vi "pitchrolldistance.vi"(11 "input":dbl[](array[numeric])) -> (3 "A * B 2":T1)   [LabVIEW 2015]
uses:
  <vilib>/Analysis/Matrix/Datatypes/RealMatrix.ctl
  <vilib>/Analysis/baseanly.llb/Unit Vector (DBL).vi
  <vilib>/Analysis/Matrix/Numeric/Conversions/Array To Matrix - RA2.vi
  <vilib>/Analysis/Matrix/Numeric/Conversions/Array To Matrix - RA.vi
  <vilib>/Analysis/Matrix/Numeric/Subtract/Subtract - RM,RM.vi
  <vilib>/Analysis/Matrix/Numeric/Multiply/Multiply - RM,RM.vi
  <vilib>/Analysis/NI_AALPro.lvlib
  <vilib>/Analysis/Matrix/NI_Matrix.lvlib
  <vilib>/Analysis/NI_AALBase.lvlib
panel:
  out "Position points":i32[][](array[numeric])
  out "Unit Vector":dbl[](array[numeric]) format="%0.2f"
  out "A * B":T1
  out "Real Matrix (Column Vector)":T1
  out "Real Matrix":T1
  out "x-y 2":dbl[](array[numeric])
  out "x-y":dbl[](array[numeric])
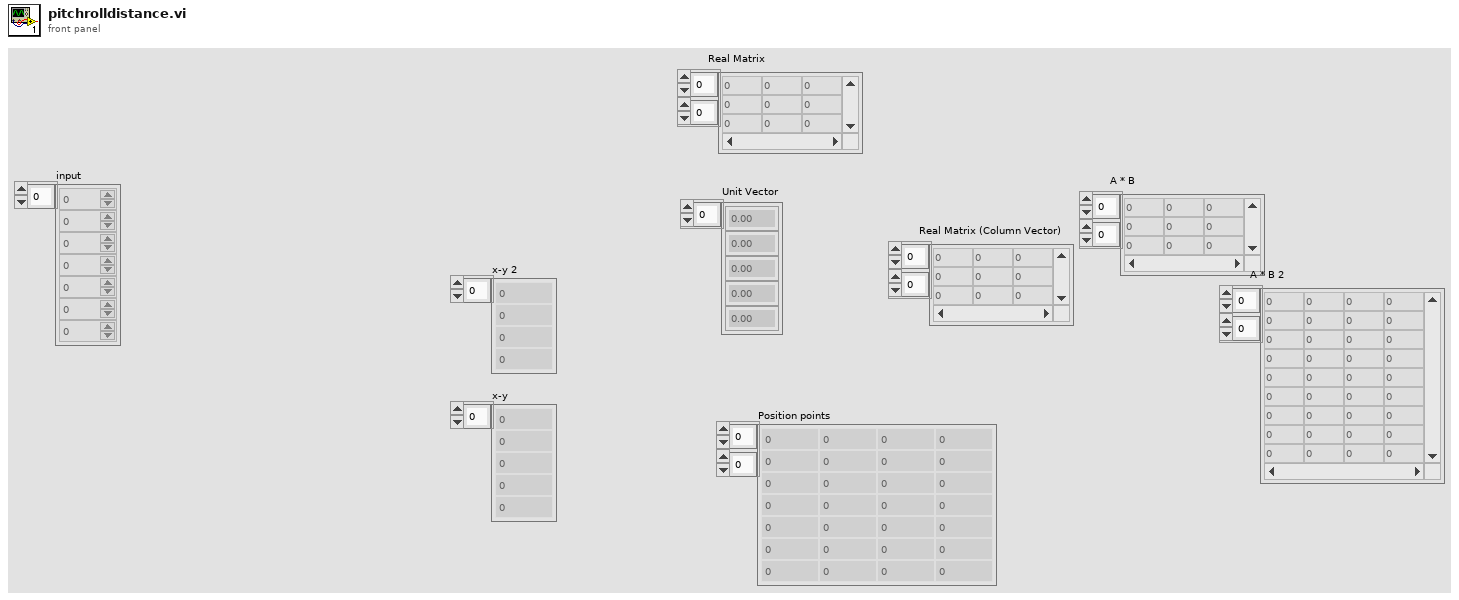
[diagram p1: front panel]
types:
  T1 = typedef "NI_Matrix.lvlib/RealMatrix.ctl" = dbl[][]
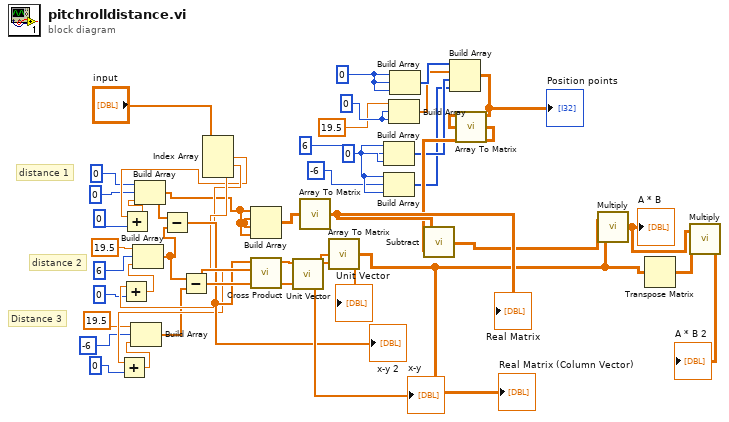
[diagram p0: block diagram]
diagram:
  w6 = 0
  w8 = 0
  w20 = 0
  # "Distance 3"
  # "distance 2"
  # "distance 1"
  n1 = Index Array(array="input") -> (element #1=w36:dbl, element #2=w37:dbl, element #3=w38:dbl)  [unwired: 3 in]
  n2 = Add(x=w38, y=0) -> (x+y=w31:dbl)
  n3 = Add(x=w37, y=0) -> (x+y=w32:dbl)
  n4 = Add(x=w36, y=0) -> (x+y=w34:dbl)
  n5 = Build Array(19.5, -6, w31) -> (w22:dbl[])
  n6 = Build Array(19.5, 6, w32) -> (w39:dbl[])
  n7 = Build Array(0, 0, w34) -> (w1:dbl[])
  n8 = Subtract(x=w1, y=w39) -> (x-y=w40:dbl[])
  "x-y 2" <- w40
  n9 = Subtract(x=w39, y=w22) -> (x-y=w41:dbl[])
  "x-y" <- w41
  n10 = Build Array(w1, w1, w1, w1) -> (w42:dbl[][])
  n11 = call <vilib>:"Cross Product.vi"("B Vector"=w41, "A Vector"=w40) -> ("Cross Product"=w10:dbl[])  [unwired: 8 in, 1 out]
  n12 = call-poly <vilib>:"Unit Vector.vi"("Input Vector"=w10) -> ("Unit Vector"=w9:dbl[])  [unwired: 8 in, 2 out]
  "Unit Vector" <- w9
  n13 = call-poly <vilib>:"Array To Matrix.vi"("Real 2D Array"=w42) -> ("Real Matrix"=w21:T1)
  "Real Matrix" <- w21
  n14 = call-poly <vilib>:"Array To Matrix.vi"("Real 1D Array"=w9) -> ("Real Matrix (Column Vector)"=w14:T1)
  "Real Matrix (Column Vector)" <- w14
  n15 = Build Array(w6, 6, w6) -> (w3:i32[])
  n16 = Build Array(w6, -6, w6) -> (w2:i32[])
  n17 = Build Array(19.5, w8, w8) -> (w18:dbl[])
  n18 = Build Array(w20, w20, w20) -> (w19:i32[])
  n19 = Build Array(w19, w18, w3, w2) -> (w17:dbl[][])
  "Position points" <- w17
  n20 = call-poly <vilib>:"Array To Matrix.vi"("Real 2D Array"=w17) -> ("Real Matrix"=w16:T1)
  n21 = call-poly <vilib>:"Subtract.vi"("Real Matrix B"=w16, "Real Matrix A"=w21) -> ("A - B"=w15:T1)
  n22 = call-poly <vilib>:"Multiply.vi"("Real Matrix B"=w14, "Real Matrix A"=w15) -> ("A * B"=w13:T1)
  "A * B" <- w13
  n23 = Transpose Matrix(1:w14) -> (0:w12:T1)
  n24 = call-poly <vilib>:"Multiply.vi"("Real Matrix B"=w12, "Real Matrix A"=w13) -> ("A * B"=→"A * B 2":T1)
